vi "Set Server gRPC UEs.vi"(10 "Server RPC Methods":T1, 11 "OOP Server in":refnum<class "Streamer_server.lvclass">) -> (3 "OOP Server out":refnum<class "Streamer_server.lvclass">)   [LabVIEW 2019, in "Streamer_server.lvlib" / "Streamer_server.lvclass"]
uses:
  Streamer_server.lvclass
  typeDefs/Server gRPC UEs.ctl
  <vilib>/gRPC/LabVIEW gRPC Library/Server API/typeDefs/gRPCId Cluster.ctl
  <vilib>/gRPC/LabVIEW gRPC Library/Server API/typeDefs/grpcId.ctl
  Streamer_server.lvclass/Streamer_server.ctl
  <vilib>/gRPC/LabVIEW gRPC Library/gprc-lvsupport-release.lvlib
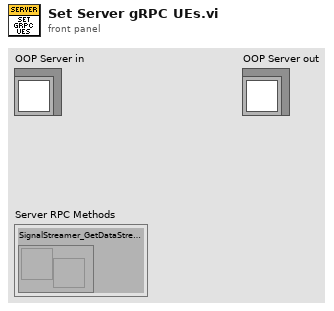
[diagram p1: front panel]
types:
  T1 = typedef "Streamer_server.lvlib/Streamer_server.lvclass/Server gRPC UEs.ctl" = cluster{"SignalStreamer_GetDataStream gRPC UE":refnum<user-event>}
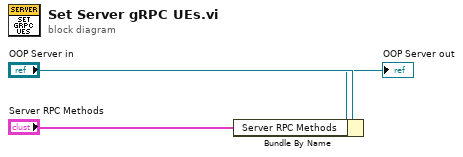
[diagram p0: block diagram]
diagram:
  n1 = Bundle By Name(cluster="OOP Server in", "Server RPC Methods"="Server RPC Methods") -> (→"OOP Server out":refnum<class "Streamer_server.lvclass">)
